vi "Get Baselines From Cursor.vi"(0 "Graph Reference":refnum<vi>) -> (1 "Force Baseline (pN)":dbl, 2 "Extension Baseline (nm)":dbl)   [LabVIEW 2013]
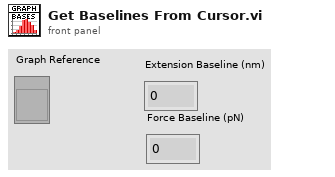
[diagram p1: front panel]
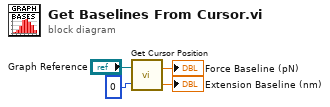
[diagram p0: block diagram]
diagram:
  n1 = call "Get Cursor Position.vi"("Cursor ID"=u32 0 ("Active Cursor"), "Graph Reference"="Graph Reference") -> ("X Position"=→"Extension Baseline (nm)":dbl, "Y Position"=→"Force Baseline (pN)":dbl)
